vi "GCSTranslateError.vi"(5 "error in":errorcluster) -> (14 "GCS Error?":bool, 15 "Error Description":string, 19 "error out":errorcluster)   [LabVIEW 2020]
doc: "Returns if error in contains a GCS error code and if this is the case, it displays the corresponding error message and appends it to \"source\" in error out."
panel:
  # "Returns if error in contains a GCS error code and if this is the \ncase, it displays the corresponding error message and \nappends it to \"source\" in \"error out\"."
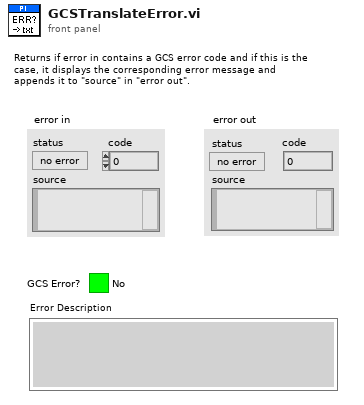
[diagram p1: front panel]
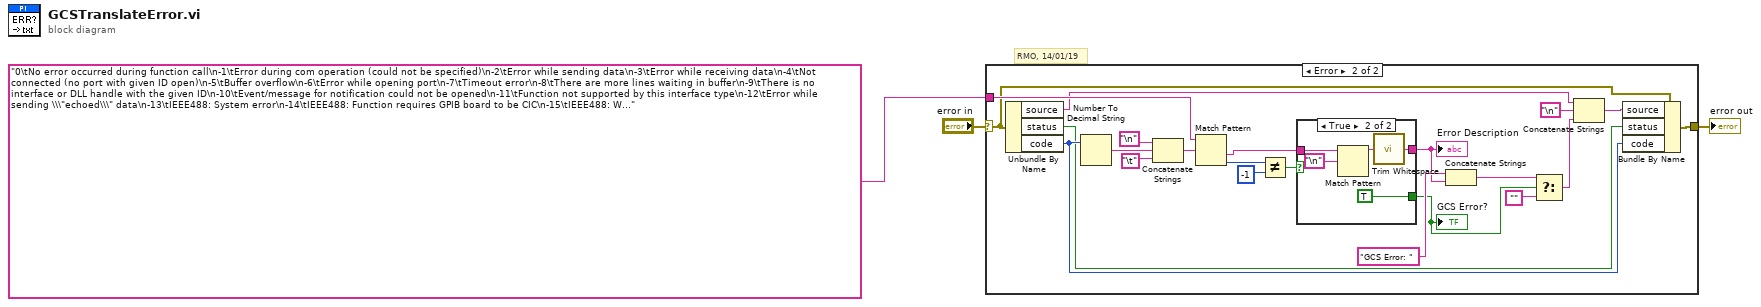
[diagram p0: block diagram]
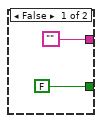
[diagram p3: hidden frame]
diagram:
  # "RMO, 14/01/19"
  n1 = case shown="Error" "error in" {
    selector: "error in" -> [w4 w6]
    tunnel: "0\tNo error occurred during function call\n-1\tError during com operation (could not be specified)\n-2\tError while sending data\n-3\tError while receiving data\n-4\tNot connected (no port with given ID open)\n-5\tBuffer overflow\n-6\tError while opening port\n-7\tTimeout error\n-8\tThere are more lines waiting in buffer\n-9\tThere is no interface or DLL handle with the given ID\n-10\tEvent/message for notification could not be opened\n-11\tFunction not supported by this interface type\n-12\tError while sending \\\"echoed\\\" data\n-13\tIEEE488: System error\n-14\tIEEE488: Function requires GPIB board to be CIC\n-15\tIEEE488: Write function detected no listeners\n-16\tIEEE488: Interface board not addressed correctly\n-17\tIEEE488: Invalid argument to function call\n-18\tIEEE488: Function requires GPIB board to be SAC\n-19\tIEEE488: I/O operation aborted\n-20\tIEEE488: Interface board not found\n-21\tIEEE488: Error performing DMA\n-22\tIEEE488: I/O operation started before previous operation completed\n-23\tIEEE488: No capability for intended operation\n-24\tIEEE488: File system operation error\n-25\tIEEE488: Command error during device call\n-26\tIEEE488: Serial poll-status byte lost\n-27\tIEEE488: SRQ remains asserted\n-28\tIEEE488: Return buffer full\n-29\tIEEE488: Address or board locked\n-30\tRS-232: 5 data bits with 2 stop bits is an invalid combination, as is 6, 7, or 8 data bits with 1.5 stop bits\n-31\tRS-232: Error configuring the COM port\n-32\tError dealing with internal system resources (events, threads, ...)\n-33\tA DLL or one of the required functions could not be loaded\n-34\tFTDIUSB: invalid handle\n-35\tFTDIUSB: device not found\n-36\tFTDIUSB: device not opened\n-37\tFTDIUSB: IO error\n-38\tFTDIUSB: insufficient resources\n-39\tFTDIUSB: invalid parameter\n-40\tFTDIUSB: invalid baud rate\n-41\tFTDIUSB: device not opened for erase\n-42\tFTDIUSB: device not opened for write\n-43\tFTDIUSB: failed to write device\n-44\tFTDIUSB: EEPROM read failed\n-45\tFTDIUSB: EEPROM write failed\n-46\tFTDIUSB: EEPROM erase failed\n-47\tFTDIUSB: EEPROM not present\n-48\tFTDIUSB: EEPROM not programmed\n-49\tFTDIUSB: invalid arguments\n-50\tFTDIUSB: not supported\n-51\tFTDIUSB: other error\n-52\tError while opening the COM port: was already open\n-53\tChecksum error in received data from COM port\n-54\tSocket not ready, you should call the function again\n-55\tPort is used by another socket\n-56\tSocket not connected (or not valid)\n-57\tConnection terminated (by peer)\n-58\tCan't connect to peer\n-59\tOperation was interrupted by a nonblocked signal\n-60\tNo Device with this ID is present\n-61\tDriver could not be opened (on Vista: run as administrator!)\n-62\tHost not found\n-63\tDevice already connected\n-1001\tUnknown axis identifier\n-1002\tNumber for NAV out of range--must be in [1,10000]\n-1003\tInvalid value for SGA--must be one of {1, 10, 100, 1000}\n-1004\tController sent unexpected response\n-1005\tNo manual control pad installed, calls to SMA and related commands are not allowed\n-1006\tInvalid number for manual control pad knob\n-1007\tAxis not currently controlled by a manual control pad\n-1008\tController is busy with some lengthy operation (e.g. reference move, fast scan algorithm)\n-1009\tInternal error--could not start thread\n-1010\tController is (already) in macro mode--command not valid in macro mode\n-1011\tController not in macro mode--command not valid unless macro mode active\n-1012\tCould not open file to write or read macro\n-1013\tNo macro with given name on controller, or macro is empty\n-1014\tInternal error in macro editor\n-1015\tOne or more arguments given to function is invalid (empty string, index out of range, ...)\n-1016\tAxis identifier is already in use by a connected stage\n-1017\tInvalid axis identifier\n-1018\tCould not access array data in COM server\n-1019\tRange of array does not fit the number of parameters\n-1020\tInvalid parameter ID given to SPA or SPA?\n-1021\tNumber for AVG out of range--must be >0\n-1022\tIncorrect number of samples given to WAV\n-1023\tGeneration of wave failed\n-1024\tMotion error: position error too large, servo is switched off automatically\n-1025\tController is (already) running a macro\n-1026\tConfiguration of PZT stage or amplifier failed\n-1027\tCurrent settings are not valid for desired configuration\n-1028\tUnknown channel identifier\n-1029\tError while reading/writing wave generator parameter file\n-1030\tCould not find description of wave form. Maybe WG.INI is missing?\n-1031\tThe WGWaveEditor DLL function was not found at startup\n-1032\tThe user cancelled a dialog\n-1033\tError from C-844 Controller\n-1034\tDLL necessary to call function not loaded, or function not found in DLL\n-1035\tThe open parameter file is protected and cannot be edited\n-1036\tThere is no parameter file open\n-1037\tSelected stage does not exist\n-1038\tThere is already a parameter file open. Close it before opening a new file\n-1039\tCould not open parameter file\n-1040\tThe version of the connected controller is invalid\n-1041\tParameter could not be set with SPA--parameter not defined for this controller!\n-1042\tThe maximum number of wave definitions has been exceeded\n-1043\tThe maximum number of wave generators has been exceeded\n-1044\tNo wave defined for specified axis\n-1045\tWave output to axis already stopped/started\n-1046\tNot all axes could be referenced\n-1047\tCould not find parameter set required by frequency relation\n-1048\tCommand ID given to SPP or SPP? is not valid\n-1049\tA stage name given to CST is not unique\n-1050\tA uuencoded file transfered did not start with \\\"begin\\\" followed by the proper filename\n-1051\tCould not create/read file on host PC\n-1052\tChecksum error when transfering a file to/from the controller\n-1053\tThe PiStages.dat database could not be found. This file is required to connect a stage with the CST command\n-1054\tNo wave being output to specified axis\n-1055\tInvalid password\n-1056\tError during communication with OPM (Optical Power Meter), maybe no OPM connected\n-1057\tWaveEditor: Error during wave creation, incorrect number of parameters\n-1058\tWaveEditor: Frequency out of range\n-1059\tWaveEditor: Error during wave creation, incorrect index for integer parameter\n-1060\tWaveEditor: Error during wave creation, incorrect index for floating point parameter\n-1061\tWaveEditor: Error during wave creation, could not calculate value\n-1062\tWaveEditor: Graph display component not installed\n-1063\tUser Profile Mode: Command is not allowed, check for required preparatory commands\n-1064\tUser Profile Mode: First target position in User Profile is too far from current position\n-1065\tController is (already) in User Profile Mode\n-1066\tUser Profile Mode: Block or Data Set index out of allowed range\n-1067\tProfileGenerator: No profile has been created yet\n-1068\tProfileGenerator: Generated profile exceeds limits of one or both axes\n-1069\tProfileGenerator: Unknown parameter ID in Set/Get Parameter command\n-1070\tProfileGenerator: Parameter out of allowed range\n-1071\tUser Profile Mode: Out of memory\n-1072\tUser Profile Mode: Cluster is not assigned to this axis\n-1073\tUnknown cluster identifier\n-1074\tThe installed device driver doesn't match the required version. Please see the documentation to determine the required device driver version.\n-1075\tThe library used doesn't match the required version. Please see the documentation to determine the required library version.\n-1076\tThe interface is currently locked by another function. Please try again later.\n-1077\tVersion of parameter DAT file does not match the required version. Current files are available at www.pi.ws.\n-1078\tCannot write to parameter DAT file to store user defined stage type.\n-1079\tCannot create parameter DAT file to store user defined stage type.\n-1080\tParameter DAT file does not have correct revision.\n-1081\tUser stages DAT file does not have correct revision.\n-1082\tTimeout Error. Some lengthy operation did not finish within expected time.\n-1083\tA function argument has an unexpected datatype.\n-1084\tLength of data arrays is different.\n-1085\tParameter value not found in parameter DAT file.\n-1086\tMacro recording is not allowed in this mode of operation.\n-1087\tcommand cancelled by user input.\n-1088\tController sent too few GCS data sets\n-1089\tController sent too many GCS data sets\n-1090\tCommunication error while reading GCS data\n-1091\tWrong number of input arguments.\n-1092\tChange of command level has failed.\n-1093\tSwitching off the servo mode has failed.\n-1094\tA parameter could not be set while performing CST: CST was not performed (parameters remain unchanged).\n-1095\tConnection could not be reestablished after reboot.\n-1096\tSending HPA? or receiving the response has failed.\n-1097\tHPA? response does not comply with GCS2 syntax.\n-1098\tResponse to SPA? could not be received.\n-1099\tVersion of PAM file cannot be handled (too old or too new)\n-1100\tPAM file does not contain required data in PAM-file format\n-1101\tInformation does not contain all required data\n-1102\tNo value for parameter available\n-1103\tNo PAM file is open\n-1104\tInvalid value\n-1105\tUnknown parameter\n-1106\tResponse to SEP? could not be received.\n-1107\tResponse to SPA? could not be received.\n-1108\tError while performing CST: One or more parameters were not set correctly.\n-1109\tPAM file has duplicate entry with different values.\n-1110\tFile has no signature\n-1111\tFile has invalid signature\n-1112\tCannot determine actual end of travel range while platform is moving.\n-1113\tSending IDN? or receiving the response has failed.\n-1114\tSending MAC_DEF or receiving the response has failed.\n-1115\tSending Controller or controller version does not exist in PIStages database.\n-1116\tNot enough memory\n-1117\tRuntime error indicated for axis, check error log with \\\"LOG?\\\" to find more details.\n-1118\tCritical error indicated for system, check error log with \\\"LOG?\\\" to find more details.\n-10000\tPI stage database: String containing stage type and description has invalid format.\n-10001\tPI stage database: Database does not contain the selected stage type for the connected controller.\n-10002\tPI stage database: Establishing the connection has failed.\n-10003\tPI stage database: Communication was interrupted (e.g. because database was deleted).\n-10004\tPI stage database: Querying data failed.\n-10005\tPI stage database: System already exists. Rename stage and try again.\n-10006\tPI stage database: Response to HPA? contains unknown parameter IDs.\n-10007\tPI stage database: Inconsistency between database and response to HPA?.\n-10008\tPI stage database: Stage has not been added.\n-10009\tPI stage database: Stage has not been removed.\n-10010\tController does not support all stage parameters stored in PI stage database. No parameters were set.\n-10011\tThe version of PISTAGES3.DB stage database is out of date. Please update via PIUpdateFinder. No parameters were set.\n-10012\tMismatch between number of parameters present in stage database and available in controller interface. No parameters were set.\n-10013\tMismatch between number of parameters present in stage database and available in controller interface. Some parameters were ignored.\n-10014\tOne or more parameters could not be set correctly on the controller.\n-10015\tOne or more parameter definitions are not present in stage database. Please update PISTAGES3.DB via PIUpdateFinder. Missing parameters were ignored.\n-10016\tParameters could not be set on controller because the corresponding firmware feature is missing\n0\tNo error\n1\tParameter syntax error\n2\tUnknown command\n3\tCommand length out of limits or command buffer overrun\n4\tError while scanning\n5\tUnallowable move attempted on unreferenced axis, or move attempted with servo off\n6\tParameter for SGA not valid\n7\tPosition out of limits\n8\tVelocity out of limits\n9\tAttempt to set pivot point while U,V and W not all 0\n10\tController was stopped by command\n11\tParameter for SST or for one of the embedded scan algorithms out of range\n12\tInvalid axis combination for fast scan\n13\tParameter for NAV out of range\n14\tInvalid analog channel\n15\tInvalid axis identifier\n16\tInvalid stage name\n17\tParameter out of range\n18\tInvalid macro name\n19\tError while recording macro\n20\tMacro not found\n21\tAxis has no brake\n22\tAxis identifier specified more than once\n23\tIllegal axis or channel\n24\tIncorrect number of parameters\n25\tInvalid floating point number\n26\tParameter missing\n27\tSoft limit out of range\n28\tNo manual pad found\n29\tNo more step-response values\n30\tNo step-response values recorded\n31\tAxis has no reference sensor\n32\tAxis has no limit switch\n33\tNo relay card installed\n34\tCommand not allowed for selected stage(s)\n35\tNo digital input installed\n36\tNo digital output configured\n37\tNo more MCM responses\n38\tNo MCM values recorded\n39\tController number invalid\n40\tNo joystick configured\n41\tInvalid axis for electronic gearing, axis can not be slave\n42\tPosition of slave axis is out of range\n43\tSlave axis cannot be commanded directly when electronic gearing is enabled\n44\tCalibration of joystick failed\n45\tReferencing failed\n46\tOPM (Optical Power Meter) missing\n47\tOPM (Optical Power Meter) not initialized or cannot be initialized\n48\tOPM (Optical Power Meter) Communication Error\n49\tMove to limit switch failed\n50\tAttempt to reference axis with referencing disabled\n51\tSelected axis is controlled by joystick\n52\tController detected communication error\n53\tCommand is not allowed while the affected axis is in motion.\n54\tUnknown parameter\n55\tNo commands were recorded with REP\n56\tPassword invalid\n57\tData recorder table does not exist\n58\tSource option does not exist; number too low or too high\n59\tSource ID (channel or axis) too low or too high\n60\tProtected Param: current Command Level (CCL) too low\n61\tCommand execution not possible while Autozero is running\n62\tAutozero requires at least one linear axis\n63\tInitialization still in progress\n64\tParameter is read-only\n65\tParameter not found in non-volatile memory\n66\tVoltage out of limits\n67\tNot enough memory available for requested wave curve\n68\tNot enough memory available for DDL table; DDL can not be started\n69\tTime delay larger than DDL table; DDL can not be started\n70\tThe requested arrays have different lengths; query them separately\n71\tAttempt to restart the generator while it is running in single step mode\n72\tMotion commands and wave generator activation are not allowed when analog target is active\n73\tMotion commands are not allowed when wave generator output is active; use WGO to disable generator output\n74\tNo sensor channel or no piezo channel connected to selected axis (sensor and piezo matrix)\n75\tGenerator started (WGO) without having selected a wave table (WSL).\n76\tInterface buffer did overrun and command couldn't be received correctly\n77\tData Record Table does not hold enough recorded data\n78\tData Record Table is not configured for recording\n79\tOpen-loop commands are not allowed when servo is on\n80\tHardware error affecting RAM\n81\tNot macro command\n82\tMacro counter out of range\n83\tJoystick is active\n84\tMotor is off\n85\tMacro-only command\n86\tInvalid joystick axis\n87\tJoystick unknown\n88\tMove without referenced stage\n89\tCommand not allowed in current motion mode\n90\tNo tracing possible while digital IOs are used on this HW revision. Reconnect to switch operation mode.\n91\tMove not possible, would cause collision\n92\tStage is not capable of following the master. Check the gear ratio(SRA).\n93\tThis command is not allowed while the affected axis or its master is in motion.\n94\tServo cannot be switched on when open-loop joystick control is enabled.\n95\tThis parameter cannot be changed in current servo mode.\n96\tUnknown stage name\n97\tInvalid length of value (too much characters)\n98\tAutoZero procedure was not successful\n99\tSensor voltage is off\n100\tPI LabVIEW driver reports error. See source control for details.\n200\tNo stage connected to axis\n201\tFile with axis parameters not found\n202\tInvalid axis parameter file\n203\tBackup file with axis parameters not found\n204\tPI internal error code 204\n205\tSMO with servo on\n206\tuudecode: incomplete header\n207\tuudecode: nothing to decode\n208\tuudecode: illegal UUE format\n209\tCRC32 error\n210\tIllegal file name (must be 8-0 format)\n211\tFile not found on controller\n212\tError writing file on controller\n213\tVEL command not allowed in DTR Command Mode\n214\tPosition calculations failed\n215\tThe connection between controller and stage may be broken\n216\tThe connected stage has driven into a limit switch, some controllers need CLR to resume operation\n217\tStrut test command failed because of an unexpected strut stop\n218\tWhile MOV! is running position can only be estimated!\n219\tPosition was calculated during MOV motion\n220\tFIFO buffer underrun during interpolation\n221\tFIFO buffer overflow during interpolation\n230\tInvalid handle\n231\tNo bios found\n232\tSave system configuration failed\n233\tLoad system configuration failed\n301\tSend buffer overflow\n302\tVoltage out of limits\n303\tOpen-loop motion attempted when servo ON\n304\tReceived command is too long\n305\tError while reading/writing EEPROM\n306\tError on I2C bus\n307\tTimeout while receiving command\n308\tA lengthy operation has not finished in the expected time\n309\tInsufficient space to store macro\n310\tConfiguration data has old version number\n311\tInvalid configuration data\n333\tInternal hardware error\n400\tWave generator index error\n401\tWave table not defined\n402\tWave type not supported\n403\tWave length exceeds limit\n404\tWave parameter number error\n405\tWave parameter out of range\n406\tWGO command bit not supported\n500\tThe \\\"red knob\\\" is still set and disables system\n501\tThe \\\"red knob\\\" was activated and still disables system - reanimation required\n502\tPosition consistency check failed\n503\tHardware collision sensor(s) are activated\n504\tStrut following error occurred, e.g. caused by overload or encoder failure\n505\tOne sensor signal is not valid\n506\tServo loop was unstable due to wrong parameter setting and switched off to avoid damage.\n507\tdigital connection to external spi slave device is lost\n508\tMove attempt not permitted due to customer or limit settings\n509\tEmergency stop caused by trigger input\n530\tA command refers to a coordinate system that does not exist\n531\tA command refers to a coordinate system that has no parent node\n532\tAttempt to delete or change a coordinate system that is in use\n533\tDefinition of a coordinate system is cyclic\n536\tCoordinate system cannot be defined as long as Hexapod is in motion\n537\tCoordinate system type is not intended for manual enabling\n539\tA coordinate system cannot be linked to itself\n540\tCoordinate system definition is erroneous or not complete (replace or delete it)\n542\tThe coordinate systems are not part of the same chain\n543\tUnused coordinate system must be deleted before new coordinate system can be stored\n544\tWith this coordinate system type SPI usage is not supported\n545\tSoft limits invalid due to changes in coordinate system\n546\tCoordinate system is write protected\n547\tCoordinate system cannot be changed because its content is loaded from a configuration file\n548\tCoordinate system may not be linked\n549\tA KSB-type coordinate system can only be rotated by multiples of 90 degrees\n551\tThis query is not supported for this coordinate system type\n552\tThis combination of work and tool coordinate systems does not exist\n553\tThe combination must consist of one work and one tool coordinate system\n554\tThis coordinate system type does not exist\n555\tBasMac: unknown controller error\n556\tNo coordinate system of this type is enabled\n557\tName of coordinate system is invalid\n558\tFile with stored CS systems is missing or erroneous\n559\tFile with leveling CS is missing or erroneous\n601\tNot enough memory\n602\tHardware voltage error\n603\tHardware temperature out of range\n604\tPosition error of any axis in the system is too high\n606\tMaximum value of input signal has been exceeded\n607\tValue is not integer\n608\tFast alignment process cannot be paused because it is not running\n609\tFast alignment process cannot be restarted/resumed because it is not paused\n650\tParameter could not be set with SPA - SEP needed?\n651\tPhase finding error\n652\tSensor setup error\n653\tSensor communication error\n654\tMotor amplifier error\n655\tOvercurrent protection triggered by I2T-module\n656\tOvercurrent protection triggered by amplifier module\n657\tSafety stop triggered\n658\tSensor off?\n659\tParameter could not be set. Conflict with another parameter.\n700\tCommand not allowed in external mode\n710\tExternal mode communication error\n715\tInvalid mode of operation\n716\tFirmware stopped by command (#27)\n717\tExternal mode driver missing\n718\tMissing or incorrect configuration of external mode\n719\tExternal mode cycletime invalid\n720\tBrake is activated\n725\tDrive state transition error\n731\tCommand not allowed while surface detection is running\n732\tLast surface detection failed\n733\tFieldbus is active and is blocking GCS control commands\n1000\tToo many nested macros\n1001\tMacro already defined\n1002\tMacro recording not activated\n1003\tInvalid parameter for MAC\n1004\tDeleting macro failed\n1005\tController is busy with some lengthy operation (e.g. reference move, fast scan algorithm)\n1006\tInvalid identifier (invalid special characters, ...)\n1007\tVariable or argument not defined\n1008\tController is (already) running a macro\n1009\tInvalid or missing operator for condition. Check necessary spaces around operator.\n1010\tNo answer was received while executing WAC/MEX/JRC/...\n1011\tCommand not valid during macro execution\n1012\tError occured during macro execution\n1013\tNo macro with given name on controller, or macro is empty\n1015\tOne or more arguments given to function is invalid (empty string, index out of range, ...)\n1024\tMotion error: position error too large, servo is switched off automatically\n1025\tMaximum motor output reached\n1028\tUnknown channel identifier\n1063\tUser Profile Mode: Command is not allowed, check for required preparatory commands\n1064\tUser Profile Mode: First target position in User Profile is too far from current position\n1065\tController is (already) in User Profile Mode\n1066\tUser Profile Mode: Block or Data Set index out of allowed range\n1071\tUser Profile Mode: Out of memory\n1072\tUser Profile Mode: Cluster is not assigned to this axis\n1073\tUnknown cluster identifier\n1090\tThere are too many open tcpip connections\n2000\tController already has a serial number\n2100\tEntered license is invalid\n4000\tSector erase failed\n4001\tFlash program failed\n4002\tFlash read failed\n4003\tHW match code missing/invalid\n4004\tFW match code missing/invalid\n4005\tHW version missing/invalid\n4006\tFW version missing/invalid\n4007\tFW update failed\n4008\tFW Parameter CRC wrong\n4009\tFW CRC wrong\n5000\tPicoCompensation scan data is not valid\n5001\tPicoCompensation is running, some actions can not be executed during scanning/recording\n5002\tGiven axis can not be defined as PPC axis\n5003\tDefined scan area is larger than the travel range\n5004\tGiven PicoCompensation type is not defined\n5005\tPicoCompensation parameter error\n5006\tPicoCompensation table is larger than maximum table length\n5100\tCommon error in Nexline firmware module\n5101\tOutput channel for Nexline can not be redefined for other usage\n5102\tMemory for Nexline signals is too small\n5103\tRNP can not be executed if axis is in closed loop\n5104\trelax procedure (RNP) needed\n5200\tAxis must be configured for this action\n5300\tFrequency analysis failed\n5301\tAnother frequency analysis is running\n6000\tInvalid preset value of absolute sensor\n6001\tError while writing to sensor\n6002\tError while reading from sensor\n6003\tChecksum error of absolute sensor\n6004\tGeneral error of absolute sensor\n6005\tOverflow of absolute sensor position\n0\tNo error\n16440\tThe given input port has already been registered in another connection\n16441\tThe given unit has already been registered to the broker\n16442\tThe connection has no input\n16443\tThe connection has no output\n16444\tThe sought connection is not registered\n16445\tThe input port is not connected\n16459\tAction not possible due to internal process running\n32793\tMotor output is limited\n32808\tController detected communication error\n32830\tData corrupted\n49154\tWrong number of arguments\n49155\tUnknown command\n49156\tUser command level too low for command access\n49157\tInvalid password\n49158\tUnknown section command\n49159\tReceived invalid ASCII character\n49161\tWrong data type\n49162\tUnknown parameter ID\n49163\tUser command level too low for parameter access\n49164\tArgument value not valid\n49165\tWrong parameter type\n49166\tArgument value out of range\n49167\tUnknown Axis ID\n49168\tMotion not possible due to active limit switch\n49169\tInvalid mode of operation\n49170\tAxis not referenced\n49171\tInvalid state of axis state machine\n49172\tTarget out of range\n49173\tAxis is disabled\n49174\tFault reaction active on axis\n49182\tWrong recorder format\n49183\tUnknown recorder ID\n49184\tData recorder is not in configuration mode\n49185\tWrong recorder trigger\n49186\tWrong start point\n49187\tWrong number of points\n49188\tData recorder is already running\n49189\tSpecified data recorder trace does not exist\n49190\tNot enough recorded data in at least one data recorder trace\n49191\tData recorder traces are not configured\n49193\tFirmware index unknown\n49210\tThe connection has no input\n49211\tThe connection has no output\n49212\tThe sought connection is not registered\n49215\tUnit type not supported\n49216\tFirmware update failed\n49217\tUnit could not be found\n49218\tContainer unit could not be found\n49219\tFunction unit could not be found\n49224\tMotion axis in fault state\n49227\tAction not possible due to internal process running\n49229\tInvalid expression\n49230\tExpression is too complex\n49231\tLink already set\n49232\tThe link index is wrong\n49233\tContainer unit input could not be found\n49234\tFunction unit input could not be found\n49235\tContainer unit output could not be found\n49236\tFunction unit output could not be found\n49237\tUnknown trigger ID\n65578\tCommunication timeout occurred\n65579\tInvalid Socket\n65599\tUnit type not supported\n65604\tNot enough memory\n65605\tFlash read failed\n65606\tNo data available\n65607\tFatal system error occurred\n65610\tTimeout occurred\n81928\tStop command\n81938\tAxis not referenced\n81943\tAxis has activated a limit switch\n81944\tOverheating protection: motor current is too high\n81946\tPosition error too large, servo is switched off automatically\n81947\tStop triggered by command or by error on another axis\n81993\tNo reference signal detected\n4177929\tWrong data type\n4177948\tThe max number of storable data recorders has been reached\n4177949\tThe given data recorder has already been registered\n4177964\tWrong unit ID format given\n4177965\tUnit not initialized\n4177966\tThe max number of storable connections has been reached\n4177967\tWrong arguments when setting a connection output\n4177968\tWrong arguments when setting a connection input\n4177969\tWrong device ID\n4177970\tWrong function ID\n4177971\tWrong proxy ID\n4177972\tConnection output index is out of range\n4177973\tFailed to register an interface in the bus gateway\n4177974\tFailed to register a device in the bus gateway\n4177975\tFailed to register a proxy in the bus gateway\n4177996\tHALT was triggered by command\n" -> [_ w22]
    tunnel: [w4 w7] -> w1
    frame No Error {
    }
    frame Error {
      n2 = Unbundle By Name(w6) -> ("source"=w10:string, "status"=w5:bool, "code"=w8:i32)
      n3 = Number To Decimal String(number=w8) -> (decimal integer string=w21:string)  [unwired: 1 out]
      n4 = Concatenate Strings("\n" ("string"), w21, "\t" ("string")) -> (w18:string)
      n5 = Match Pattern(string=w22, regular expression=w18) -> (after substring=w17:string, offset past match=w15:i32)  [unwired: 3 out]
      n6 = Not Equal?(x=w15, y=-1) -> (x != y?=w13:bool)
      n7 = case shown="True" w13 {
        tunnel: w17 -> [_ w33]
        tunnel: ["" w29] -> w16
        tunnel: [FALSE TRUE] -> w12
        frame False {
        }
        frame True {
          n8 = Match Pattern(string=w33, regular expression="\n" ("string")) -> (before substring=w31:string)  [unwired: 4 out]
          n9 = call "Trim Whitespace.vi"("string"=w31) -> ("trimmed string"=w29:string)  [unwired: 1 in]
        }
      }
      "Error Description" <- w16
      "GCS Error?" <- w12
      n10 = Concatenate Strings("GCS Error: " ("Substring"), w16) -> (w24:string)
      n11 = Select(t=w24, s=w12, f="") -> (s? t:f=w23:string)
      n12 = Concatenate Strings(w10, "\n", w23) -> (w9:string)
      n13 = Bundle By Name(cluster=w6, "source"=w9, "status"=w5, "code"=w8) -> (w7:errorcluster)
    }
  }
  "error out" <- w1
